vi "Save Screenshot.vi"(8 "error in (no error)":errorcluster, 10 "Screen Shot Path":path, 11 "PXIe5105 in":refnum<class "PXIe5105.lvclass">) -> (0 "error out":errorcluster, 3 "PXIe5105 out":refnum<class "PXIe5105.lvclass">)   [LabVIEW 2018, in "PXIe5105.lvlib" / "PXIe5105.lvclass"]
doc: "This Override method is used to save a screen shot of the Oscope screen."
uses:
  PXIe5105.lvclass
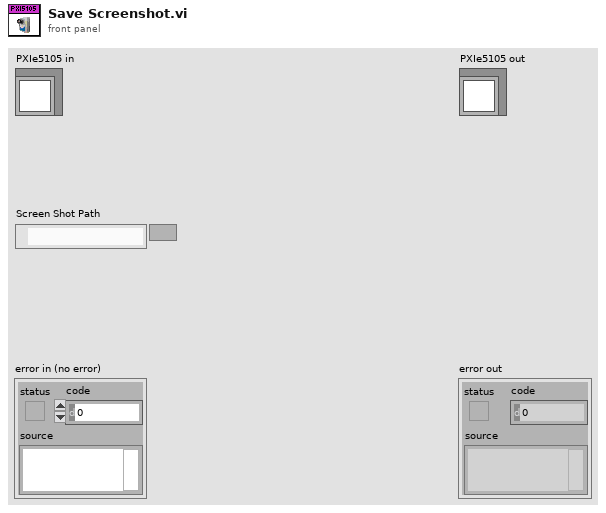
[diagram p1: front panel]
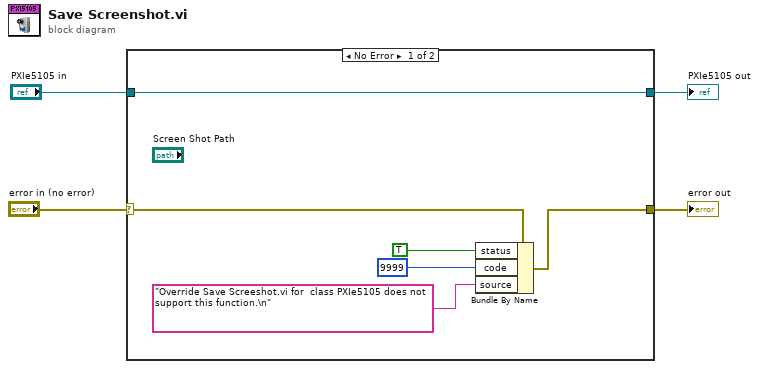
[diagram p0: block diagram]
diagram:
  n1 = case shown="No Error" "error in (no error)" {
    selector: "error in (no error)" -> [w9 w12]
    tunnel: [w5 w12] -> w3
    tunnel: "PXIe5105 in" -> [w10 w11]
    tunnel: [w10 w11] -> w1
    frame No Error {
      n2 = Bundle By Name(cluster=w9, "status"=TRUE, "code"=9999, "source"="Override Save Screeshot.vi for  class PXIe5105 does not support this function.\n") -> (w5:errorcluster)
    }
    frame Error {
    }
  }
  "error out" <- w3
  "PXIe5105 out" <- w1
